vi "Self Test.vi"(8 "error in (no error)":errorcluster, 11 "Agilent 33210A in":refnum<class "Agilent 33210A.lvclass">) -> (0 "error out":errorcluster, 3 "Agilent 33210A out":refnum<class "Agilent 33210A.lvclass">)   [LabVIEW 2021, in "Func Generator.lvlib" / "Agilent 33210A.lvclass"]
uses:
  Agilent 33210A.lvclass
  Agilent 33210A.lvclass/Agilent 33210A.ctl
  <instrlib>/Agilent 34401/Agilent 34401.lvlib
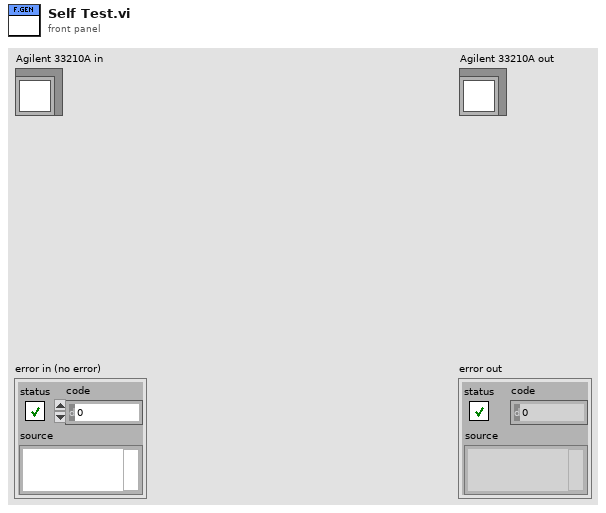
[diagram p1: front panel]
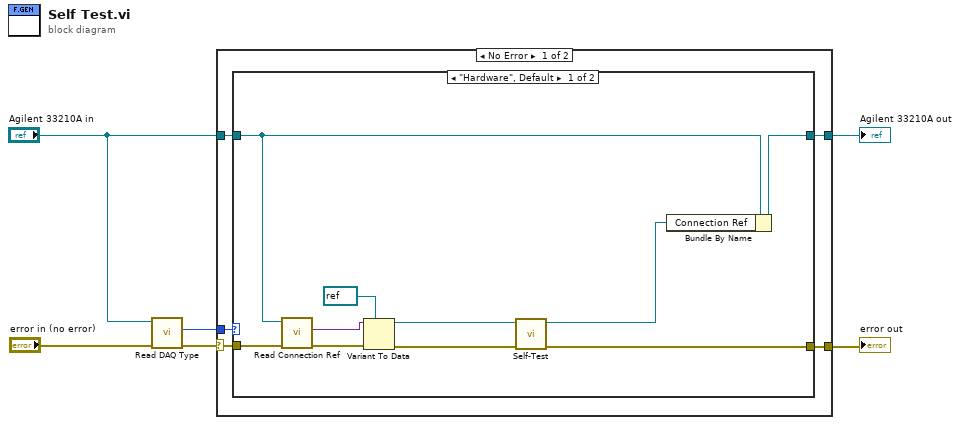
[diagram p0: block diagram]
diagram:
  n1 = call-dynamic "Read DAQ Type.vi"("error in (no error)"="error in (no error)", "Agilent 33210A in"="Agilent 33210A in") -> ("error out"=w5:errorcluster, "DAQ Type"=w4:enum16{"Hardware", "Simulation"})  [unwired: 7 in, 1 out]
  n2 = case shown="No Error" w5 {
    selector: w5 -> [w11 w24]
    tunnel: w4 -> [w10 _]
    tunnel: "Agilent 33210A in" -> [w9 w25]
    tunnel: [w8 w25] -> w2
    tunnel: [w7 w24] -> w1
    frame No Error {
      n3 = case shown="\"Hardware\", Default" w10 {
        tunnel: w11 -> [w21 w22]
        tunnel: w9 -> [w16 w23]
        tunnel: [w15 w23] -> w8
        tunnel: [w12 w22] -> w7
        frame "Hardware", Default {
          n4 = call-dynamic "Read Connection Ref.vi"("error in (no error)"=w21, "Agilent 33210A in"=w16) -> ("error out"=w20:errorcluster, "Connection Ref"=w19:variant)  [unwired: 7 in, 1 out]
          n5 = Variant To Data(error in=w20, type=refnum<visa-resource-name> refnum ("VISA resource name"), Variant=w19) -> (data=w13:refnum<visa-resource-name>, error out=w17:errorcluster)
          n6 = call <instrlib>:"Self-Test.vi"("error in (no error)"=w17, "VISA resource name"=w13) -> ("error out"=w12:errorcluster, "VISA resource name out"=w14:refnum<visa-resource-name>)  [unwired: 6 in, 2 out]
          n7 = Bundle By Name(cluster=w16, "Connection Ref"=w14) -> (w15:refnum<class "Agilent 33210A.lvclass">)
        }
        frame "Simulation" {
        }
      }
    }
    frame Error {
    }
  }
  "error out" <- w1
  "Agilent 33210A out" <- w2
